vi "Create FGV.vi"(6 "Variant in":variant, 7 "Shift Pressed?":bool, 8 "error in (no error)":errorcluster, 10 "QD Combo Box Ref":refnum<vi>, 11 "QD Launch VI Ref":refnum<vi>) -> (0 "error out":errorcluster, 4 "Variant out":variant)   [LabVIEW 2012]
doc: "PLUGIN_DESCRIPTION: \nCreate a FGV base on wire, control, indicator or constante datatype you select.\n2 FGV Templates are available: a classic FGV and a RT FGV what is made to be skipable (please see Template FGV folder)\nPLUGIN_DEFAULT_SHORTCUT: E"
uses:
  <vilib>/Utility/traverseref.llb/TRef TravTarget.ctl
  <vilib>/Utility/traverseref.llb/VI Scripting - Traverse.lvlib
panel:
  in  "Undo Name":string="Quick Drop Keyboard Shortcut"
  # "Do not change the connector pane of this VI.\n\nSee the block diagram for directions on how to use this template."
  # "Specify the name of the Undo transaction"
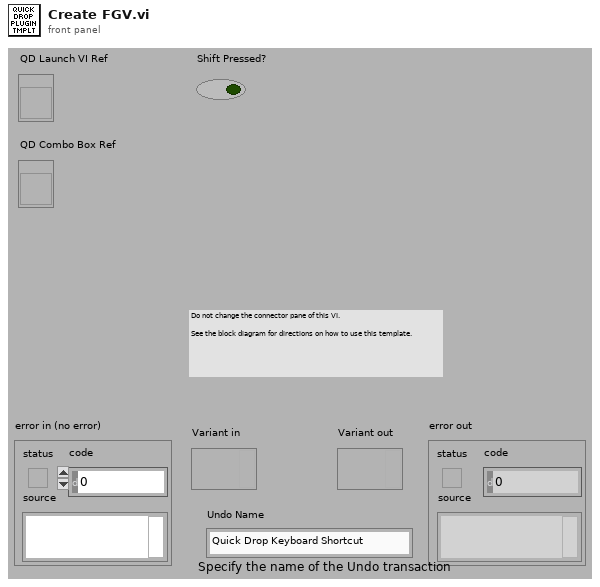
[diagram p1: front panel]
types:
  T1 = typedef "TRef TravTarget.ctl" = enum16{"FP", "BD", "Other"}
  T2 = enum32{"invalid VI type", "Standard VI", "Control VI", "Global VI", "Polymorphic VI", "Configuration VI", "SubSystem", "Facade VI", "Method VI", "Statechart Diagram VI"}
  T3 = enum32{"not a typedef", "typedef", "strict typedef", "class private data"}
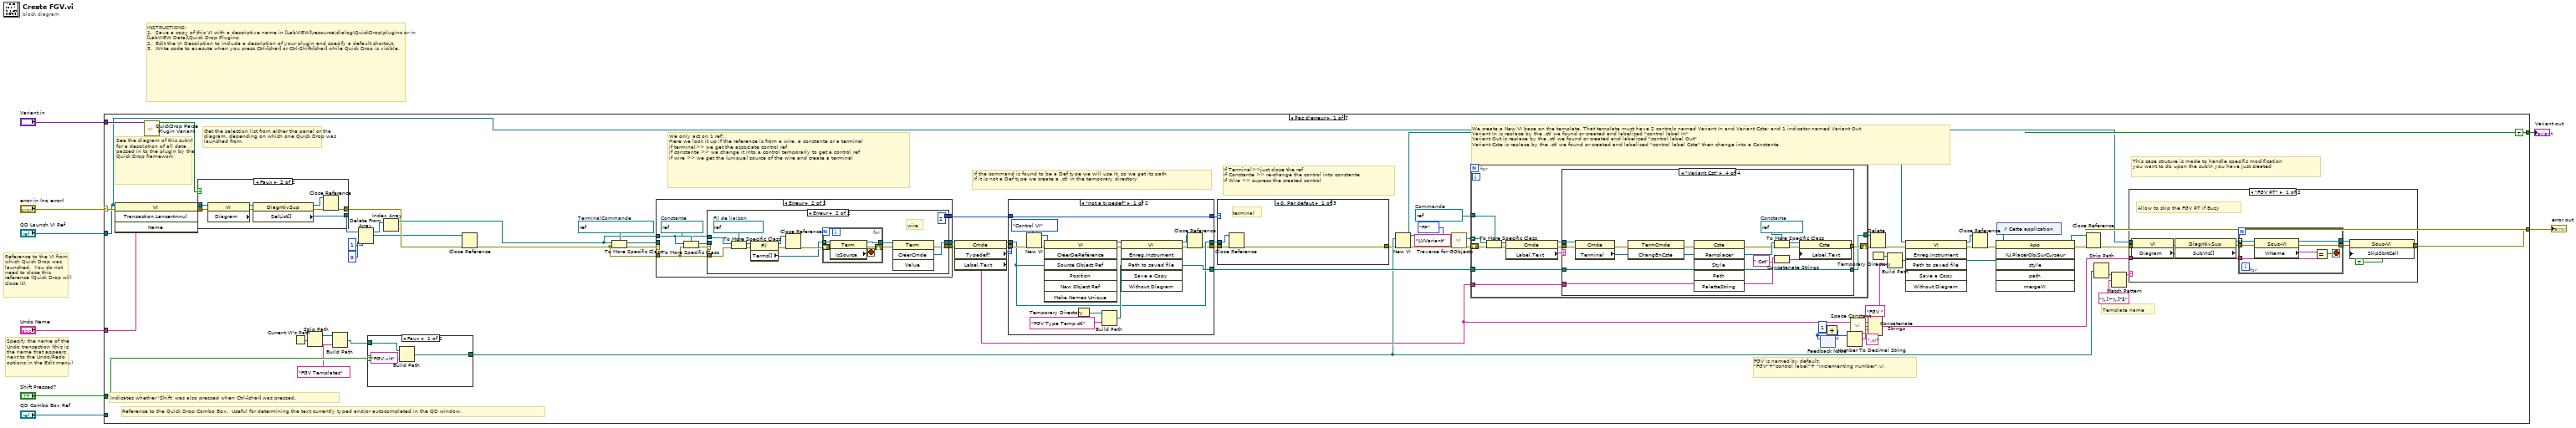
[diagram p0: block diagram]
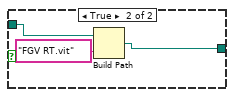
[diagram p2: hidden frame]
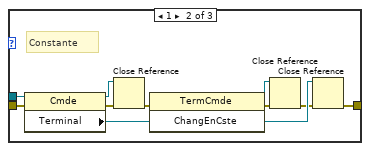
[diagram p4: hidden frame]
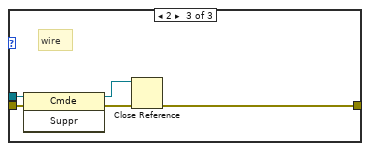
[diagram p5: hidden frame]
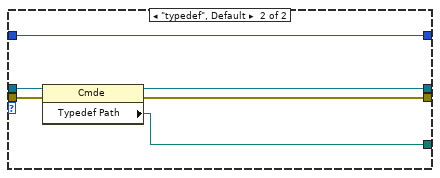
[diagram p6: hidden frame]
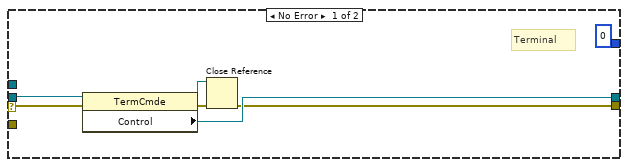
[diagram p7: hidden frame]
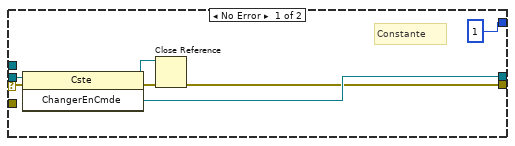
[diagram p8: hidden frame]
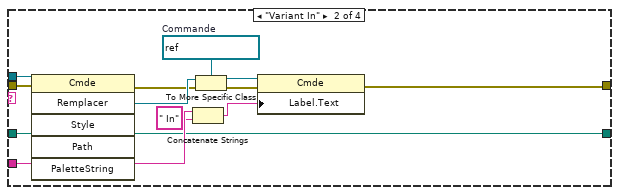
[diagram p10: hidden frame]
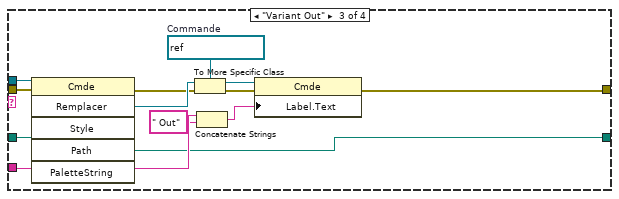
[diagram p11: hidden frame]
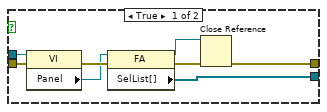
[diagram p12: hidden frame]
diagram:
  # "Specify the name of the Undo transaction (this is the name that appears next to the Undo/Redo options in the Edit menu)"
  # "Reference to the VI from which Quick Drop was launched.  You do not need to close this reference (Quick Drop will close it)."
  # "INSTRUCTIONS:\n1.  Save a copy of this VI with a descriptive name in [LabVIEW]\\resource\\dialog\\QuickDrop\\plugins or in [LabVIEW Data]\\Quick Drop Plugins.\n2.  Edit the VI Description to include a description of your plugin and specify a default shortcut. \n3.  Write code to execute when you press Ctrl-[char] or Ctrl-Shift-[char] while Quick Drop is visible."
  n1 = case shown="Pas d'erreur" "error in (no error)" {
    selector: "error in (no error)" -> [w75 w252]
    tunnel: [w16 w252] -> w7
    tunnel: "QD Launch VI Ref" -> [w23 _]
    tunnel: "Shift Pressed?" -> [w22 _]
    tunnel: "QD Combo Box Ref" -> [_ _]
    tunnel: "Variant in" -> [w76 _]
    tunnel: "Undo Name" -> [w74 _]
    tunnel: [TRUE _] -> w1
    frame No Error {
      w62 = refnum<vi> refnum  # TerminalCommande
      w64 = refnum<vi> refnum  # Commande
      # "Template name"
      # "This case struture is made to handle specific modification \nyou want to do upon the subVI you have just created"
      # "FGV is named by default:\n\"FGV\"+\"control label\"+ \"incrementing number\".vi"
      # "We create a New VI base on the template. That template must have 2 controls named Variant In and Variant Cste; and 1 indicator named Variant Out\nVariant In is replace by the .ctl we found or created and labelized \"control label In\"\nVariant Out is replace by the .ctl we found or created and labelized \"control label Out\"\nVariant Cste is replace by the .ctl we found or created and labelized \"control label Cste\" then change into a Constante"
      # "If Terminal>>just close the ref\nIf Constante >> re-change the control into constante\nIf Wire >> supress the created control"
      # "If the command is found to be a Def type we will use it, so we get its path\nIf it is not a Def type we create a .ctl in the temporary directory"
      # "We only act on 1 ref!\nHere we look it up if the reference is from a wire, a constante or a terminal\nif terminal>> we get the associate control ref \nif constante >> we change it into a control temporarly to get a control ref\nif wire >> we get the (unique) source of the wire and create a terminal"
      # "Get the selection list from either the panel or the diagram, depending on which one Quick Drop was launched from."
      # "See the diagram of this subVI for a description of all data passed in to the plugin by the Quick Drop framework"
      # "Reference to the Quick Drop Combo Box.  Useful for determining the text currently typed and/or autocompleted in the QD window."
      # "Indicates whether 'Shift' was also pressed when Ctrl-[char] was pressed."
      n2 = invoke class="VI" method="Transaction.LancerAnnul"(reference=w23, error in=w75, "Name"=w74) -> (reference out=w70:refnum<vi>, error out=w71:errorcluster)  [unwired: 1 in, 2 out]
      n3 = call <vilib>:"QuickDrop Parse Plugin Variant.vi"("QDKS Variant in"=w76) -> ("QD Launch VI Panel?"=w72:bool)  [unwired: 12 in, 2 out]
      n4 = case shown="Faux" w72 {
        tunnel: w71 -> [w243 w251]
        tunnel: w70 -> [w242 w250]
        tunnel: [w237 w245] -> w12
        tunnel: [w236 w244] -> w13
        frame True {
          n5 = property class="VI"(reference=w242, error in=w243) -> (error out=w241:errorcluster, "Panel"=w240:refnum<vi>)  [unwired: 1 out]
          n6 = property class="FA"(reference=w240, error in=w241) -> (reference out=w238:refnum<vi>, error out=w239:errorcluster, "SelList[]"=w236:refnum<vi>[])
          n7 = Close Reference(reference=w238, error in (no error)=w239) -> (error out=w237:errorcluster)
        }
        frame False {
          n8 = property class="VI"(reference=w250, error in=w251) -> (error out=w249:errorcluster, "Diagram"=w248:refnum<vi>)  [unwired: 1 out]
          n9 = property class="DiagrNivSup"(reference=w248, error in=w249) -> (reference out=w246:refnum<vi>, error out=w247:errorcluster, "SelList[]"=w244:refnum<vi>[])
          n10 = Close Reference(reference=w246, error in (no error)=w247) -> (error out=w245:errorcluster)
        }
      }
      n11 = Current VI's Path() -> (path=w21:path)
      n12 = Strip Path(path=w21) -> (stripped path=w20:path)  [unwired: 1 out]
      n13 = Build Path(base path=w20, name or relative path="FGV Templates" ("nom ou chemin relatif")) -> (appended path=w18:path)
      n14 = Delete From Array(array=w13, length=1 ("longueur"), index=0 ("indice")) -> (deleted portion=w9:refnum<vi>[], array with subset deleted=w10:refnum<vi>[])
      n15 = case shown="Faux" w22 {
        tunnel: w18 -> [w79 w82]
        tunnel: [w77 w80] -> w17
        frame False {
          n16 = Build Path(base path=w79, name or relative path="FGV.vit" ("nom ou chemin relatif")) -> (appended path=w77:path)
        }
        frame True {
          n17 = Build Path(base path=w82, name or relative path="FGV RT.vit" ("nom ou chemin relatif")) -> (appended path=w80:path)
        }
      }
      n18 = Index Array(array=w10) -> (element=w24:refnum<vi>)  [unwired: 1 in]
      n19 = Close Reference(reference=w9, error in (no error)=w12) -> (error out=w11:errorcluster)
      n20 = To More Specific Class(target class=w62, reference=w24, error in=w11) -> (specific class reference=w60:refnum<vi>, error out=w61:errorcluster)
      n21 = case shown="Erreur" w61 {
        selector: w61 -> [w145 _]
        tunnel: w60 -> [w147 _]
        tunnel: [w146 w152] -> w57
        tunnel: [w142 w151] -> w59
        tunnel: w24 -> [_ w150]
        tunnel: [0 w149] -> w51
        tunnel: w11 -> [_ w148]
        frame No Error {
          # "Terminal"
          n22 = property class="TermCmde"(reference=w147, error in=w145) -> (reference out=w141:refnum<vi>, error out=w143:errorcluster, "Control"=w146:refnum<vi>)
          n23 = Close Reference(reference=w141, error in (no error)=w143) -> (error out=w142:errorcluster)
        }
        frame Error {
          w155 = refnum<vi> refnum  # Constante
          n24 = To More Specific Class(target class=w155, reference=w150, error in=w148) -> (specific class reference=w153:refnum<vi>, error out=w154:errorcluster)
          n25 = case shown="Erreur" w154 {
            selector: w154 -> [w160 _]
            tunnel: w153 -> [w162 _]
            tunnel: [w161 w173] -> w152
            tunnel: [w156 w163] -> w151
            tunnel: w150 -> [_ w169]
            tunnel: [1 2] -> w149
            tunnel: w148 -> [_ w167]
            frame No Error {
              # "Constante"
              n26 = invoke class="Cste" method="ChangerEnCmde"(reference=w162, error in=w160) -> (reference out=w158:refnum<vi>, error out=w157:errorcluster, "Change to Control"=w161:refnum<vi>)  [unwired: 1 in]
              n27 = Close Reference(reference=w158, error in (no error)=w157) -> (error out=w156:errorcluster)
            }
            frame Error {
              w176 = refnum<vi> refnum  # Fil de liaison
              # "wire"
              n28 = To More Specific Class(target class=w176, reference=w169, error in=w167) -> (specific class reference=w175:refnum<vi>, error out=w172:errorcluster)
              n29 = property class="Fil"(reference=w175, error in=w172) -> (reference out=w165:refnum<vi>, error out=w171:errorcluster, "Terms[]"=w164:refnum<vi>[])
              n30 = Close Reference(reference=w165, error in (no error)=w171) -> (error out=w166:errorcluster)
              n31 = for {
                tunnel: w164 -> [w181] mode=indexing
                tunnel: [w180] -> w174
                shift-right: [w177] -> w170
                shift-left: w166 -> [w178]
                stop <- w179 stop-if-true
                n32 = property class="Term"(reference=w181, error in=w178) -> (reference out=w180:refnum<vi>, error out=w177:errorcluster, "IsSource"=w179:bool)
              }
              n33 = invoke class="Term" method="CréerCmde"(reference=w174, error in=w170) -> (error out=w163:errorcluster, "Create Control"=w173:refnum<vi>)  [unwired: 2 in, 2 out]
            }
          }
        }
      }
      n34 = property class="Cmde"(reference=w57, error in=w59) -> (reference out=w52:refnum<vi>, error out=w58:errorcluster, "Typedef?"=w30:T3, "Label.Text"=w47:string)
      n35 = case shown="\"not a typedef\"" w30 {
        tunnel: [w134 w139] -> w63
        tunnel: w58 -> [w124 w140]
        tunnel: w52 -> [w122 w138]
        tunnel: w51 -> [w123 w137]
        tunnel: [w123 w137] -> w50
        tunnel: [w122 w136] -> w49
        tunnel: [w121 w135] -> w40
        frame "not a typedef" {
          n36 = New VI(8:w124, 9:T2."Control VI" ("type de VI (VI standard)")) -> (0:w130:errorcluster, 3:w128:refnum<vi>)  [unwired: 5 in]
          n37 = invoke class="VI" method="CréerDeRéférence"(reference=w128, error in=w130, "Source Object Ref"=w122) -> (reference out=w129:refnum<vi>, error out=w127:errorcluster)  [unwired: 4 in, 5 out]
          n38 = Temporary Directory() -> (w132:path)
          n39 = Build Path(base path=w132, name or relative path="FGV Type Temp.ctl" ("nom ou chemin relatif")) -> (appended path=w134:path)
          n40 = invoke class="VI" method="Enreg.Instrument"(reference=w129, error in=w127, "Path to saved file"=w134) -> (reference out=w125:refnum<vi>, error out=w126:errorcluster)  [unwired: 3 in, 4 out]
          n41 = Close Reference(reference=w125, error in (no error)=w126) -> (error out=w121:errorcluster)
        }
        frame "typedef", Default {
          n42 = property class="Cmde"(reference=w138, error in=w140) -> (reference out=w136:refnum<vi>, error out=w135:errorcluster, "Typedef Path"=w139:path)
        }
      }
      n43 = case shown="0, Par défaut" w50 {
        tunnel: w49 -> [w103 w115 w120]
        tunnel: w40 -> [w104 w105 w119]
        tunnel: [w102 w106 w116] -> w34
        frame 0, Default {
          # "terminal"
          n44 = Close Reference(reference=w103, error in (no error)=w104) -> (error out=w102:errorcluster)
        }
        frame 1 {
          # "Constante"
          n45 = property class="Cmde"(reference=w115, error in=w105) -> (reference out=w112:refnum<vi>, error out=w113:errorcluster, "Terminal"=w114:refnum<vi>)
          n46 = Close Reference(reference=w112, error in (no error)=w113) -> (error out=w109:errorcluster)
          n47 = invoke class="TermCmde" method="ChangEnCste"(reference=w114, error in=w109) -> (reference out=w110:refnum<vi>, error out=w111:errorcluster, "Change To Constant"=w108:refnum<vi>)  [unwired: 1 in]
          n48 = Close Reference(reference=w110, error in (no error)=w111) -> (error out=w107:errorcluster)
          n49 = Close Reference(reference=w108, error in (no error)=w107) -> (error out=w106:errorcluster)
        }
        frame 2 {
          # "wire"
          n50 = invoke class="Cmde" method="Suppr"(reference=w120, error in=w119) -> (reference out=w117:refnum<vi>, error out=w118:errorcluster)  [unwired: 1 in, 1 out]
          n51 = Close Reference(reference=w117, error in (no error)=w118) -> (error out=w116:errorcluster)
        }
      }
      n52 = New VI(8:w34, 10:w17) -> (0:w66:errorcluster, 3:w54:refnum<vi>)  [unwired: 5 in]
      n53 = call <vilib>:"Traverse for GObjects.vi"("Traverse Target"=TRef_TravTarget."FP", "error in (no error)"=w66, "Class Name"="LVVariant", "VI Refnum"=w54) -> ("error out"=w65:errorcluster, "References"=w67:refnum<vi>[])  [unwired: 4 in, 2 out]
      n54 = for {
        tunnel: w67 -> [w193] mode=indexing
        tunnel: w64 -> [w192]
        tunnel: w63 -> [w185]
        tunnel: w47 -> [w183]
        tunnel: [w182] -> w41
        shift-right: [w184] -> w43
        shift-left: w65 -> [w191]
        n55 = To More Specific Class(target class=w192, reference=w193, error in=w191) -> (specific class reference=w190:refnum<vi>, error out=w189:errorcluster)
        n56 = property class="Cmde"(reference=w190, error in=w189) -> (reference out=w187:refnum<vi>, error out=w186:errorcluster, "Label.Text"=w188:string)
        n57 = case shown="\"Variant Cst\"" w188 {
          tunnel: w187 -> [_ w207 w219 w235]
          tunnel: w186 -> [w194 w206 w218 w233]
          tunnel: w185 -> [w195 w204 w216 w229]
          tunnel: [w194 w196 w208 w231] -> w184
          tunnel: w183 -> [_ w205 w217 w230]
          tunnel: [w195 w204 w216 w229] -> w182
          frame "", Default {
          }
          frame "Variant In" {
            w200 = refnum<vi> refnum  # Commande
            n58 = invoke class="Cmde" method="Remplacer"(reference=w207, error in=w206, "Path"=w204) -> (error out=w197:errorcluster, "Replace"=w199:refnum<vi>)  [unwired: 3 in, 4 out]
            n59 = Concatenate Strings(w205, " In" ("chaîne")) -> (w203:string)
            n60 = To More Specific Class(target class=w200, reference=w199, error in=w197) -> (specific class reference=w198:refnum<vi>, error out=w201:errorcluster)
            n61 = property class="Cmde"(reference=w198, error in=w201, "Label.Text"=w203) -> (error out=w196:errorcluster)  [unwired: 1 out]
          }
          frame "Variant Out" {
            w213 = refnum<vi> refnum  # Commande
            n62 = invoke class="Cmde" method="Remplacer"(reference=w219, error in=w218, "Path"=w216) -> (error out=w209:errorcluster, "Replace"=w210:refnum<vi>)  [unwired: 3 in, 4 out]
            n63 = To More Specific Class(target class=w213, reference=w210, error in=w209) -> (specific class reference=w212:refnum<vi>, error out=w211:errorcluster)
            n64 = Concatenate Strings(w217, " Out" ("chaîne")) -> (w215:string)
            n65 = property class="Cmde"(reference=w212, error in=w211, "Label.Text"=w215) -> (error out=w208:errorcluster)  [unwired: 1 out]
          }
          frame "Variant Cst" {
            w226 = refnum<vi> refnum  # Constante
            n66 = property class="Cmde"(reference=w235, error in=w233) -> (error out=w222:errorcluster, "Terminal"=w234:refnum<vi>)  [unwired: 1 out]
            n67 = invoke class="TermCmde" method="ChangEnCste"(reference=w234, error in=w222) -> (error out=w221:errorcluster, "Change To Constant"=w232:refnum<vi>)  [unwired: 1 in, 1 out]
            n68 = invoke class="Cste" method="Remplacer"(reference=w232, error in=w221, "Path"=w229) -> (error out=w220:errorcluster, "Replace"=w225:refnum<vi>)  [unwired: 3 in, 4 out]
            n69 = To More Specific Class(target class=w226, reference=w225, error in=w220) -> (specific class reference=w224:refnum<vi>, error out=w223:errorcluster)
            n70 = Concatenate Strings(w230, " Cst" ("chaîne")) -> (w228:string)
            n71 = property class="Cste"(reference=w224, error in=w223, "Label.Text"=w228) -> (error out=w231:errorcluster)  [unwired: 1 out]
          }
        }
      }
      n72 = feedback #1() -> (w33:u32)  [unwired: 1 in]
      n73 = Add(x=u32 1, y=w33) -> (x+y=w32:u32)
      n74 = feedback-in #1(w32) -> ()
      n75 = Number To Decimal String(number=w33) -> (decimal integer string=w45:string)  [unwired: 1 in]
      n76 = call <vilib>:"Space Constant.vi"() -> ("String"=w44:string)
      n77 = Concatenate Strings("FGV " ("chaîne"), w47, w44, w45, ".vi" ("chaîne")) -> (w25:string)
      n78 = Delete(path (use dialog)=w41, error in=w43) -> (error out=w42:errorcluster)  [unwired: 3 in, 2 out]
      n79 = Temporary Directory() -> (w53:path)
      n80 = Build Path(base path=w53, name or relative path=w25) -> (appended path=w55:path)
      n81 = invoke class="VI" method="Enreg.Instrument"(reference=w54, error in=w42, "Path to saved file"=w55) -> (reference out=w39:refnum<vi>, error out=w38:errorcluster)  [unwired: 3 in, 4 out]
      n82 = Close Reference(reference=w39, error in (no error)=w38) -> (error out=w37:errorcluster)
      n83 = control-ref of="Cette application"() -> (w56:refnum<vi>)
      n84 = invoke class="App" method="IU.PlacerObjSurCurseur"(reference=w56, error in=w37, "path"=w55) -> (reference out=w36:refnum<vi>, error out=w35:errorcluster)  [unwired: 3 in, 4 out]
      n85 = Close Reference(reference=w36, error in (no error)=w35) -> (error out=w26:errorcluster)
      n86 = Strip Path(path=w17) -> (name=w28:string)  [unwired: 1 out]
      n87 = Match Pattern(string=w28, regular expression="\\.[~\\.]*$") -> (before substring=w27:string)  [unwired: 4 out]
      n88 = case shown="\"FGV RT\"" w27 {
        tunnel: w23 -> [w92 _]
        tunnel: w25 -> [w90 _]
        tunnel: w26 -> [w87 w101]
        tunnel: [w83 w101] -> w16
        frame "FGV RT" {
          # "Allow to skip the FGV RT if Busy"
          n89 = property class="VI"(reference=w92, error in=w87) -> (error out=w86:errorcluster, "Diagram"=w93:refnum<vi>)  [unwired: 1 out]
          n90 = property class="DiagrNivSup"(reference=w93, error in=w86) -> (error out=w85:errorcluster, "SubVIs[]"=w91:refnum<vi>[])  [unwired: 1 out]
          n91 = for {
            tunnel: w91 -> [w100] mode=indexing
            tunnel: w90 -> [w98]
            tunnel: [w96] -> w89
            tunnel: w85 -> [w95]
            tunnel: [w94] -> w84
            stop <- w97 stop-if-true
            n92 = property class="Sous-VI"(reference=w100, error in=w95) -> (reference out=w96:refnum<vi>, error out=w94:errorcluster, "VIName"=w99:string)
            n93 = Equal?(x=w99, y=w98) -> (x = y?=w97:bool)
          }
          n94 = property class="Sous-VI"(reference=w89, error in=w84, "SkipSbrtCall"=TRUE ("Ignorer l'appel au sous-programme si occupé")) -> (error out=w83:errorcluster)  [unwired: 1 out]
        }
        frame "FGV", Default {
          # "Nothing specific for instance"
        }
      }
    }
    frame Error {
    }
  }
  "error out" <- w7
  "Variant out" <- w1
